vi "Get Processor Architecture.vi"() -> (0 "Processor Architecture":T1)   [LabVIEW 2020, in "binary_installation_tools.lvlib"]
uses:
  binary_installation_tools.lvlib
  <vilib>/registry/registry.llb/Registry RtKey.ctl
  <vilib>/registry/registry.llb/Registry SAM.ctl
  <vilib>/registry/registry.llb/Read Registry Value Simple STR.vi
  Processor Architecture.ctl
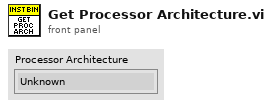
[diagram p1: front panel]
types:
  T1 = typedef "binary_installation_tools.lvlib/Processor Architecture.ctl" = enum16{"Unknown", "x86", "x64", "arm", "arm64"}
  T2 = typedef "Registry SAM.ctl" = enum32{"KEY_QUERY_VALUE", "KEY_SET_VALUE", "KEY_CREATE_SUB_KEY", "KEY_ENUMERATE_SUB_KEYS", "KEY_NOTIFY", "KEY_CREATE_LINK", "KEY_READ", "KEY_WRITE", "KEY_ALL_ACCESS", "KEY_READ | KEY_WRITE"}
  T3 = typedef "Registry RtKey.ctl" = enum32{"HKEY_CLASSES_ROOT", "HKEY_CURRENT_USER", "HKEY_LOCAL_MACHINE", "HKEY_USERS", "HKEY_PERFORMANCE_DATA", "HKEY_CURRENT_CONFIG", "HKEY_DYN_DATA"}
  T4 = typedef "Registry refnum.ctl" = refnum<k1>
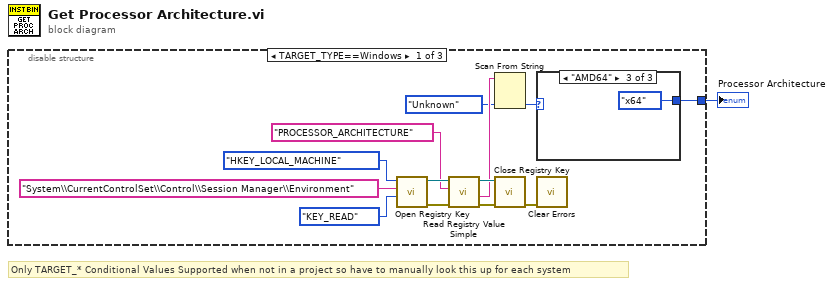
[diagram p0: block diagram]
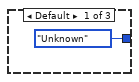
[diagram p2: hidden frame]
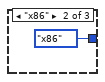
[diagram p3: hidden frame]
diagram:
  # "Only TARGET_* Conditional Values Supported when not in a project so have to manually look this up for each system"
  n1 = disable-structure shown="TARGET_TYPE==Windows" {
    disable-tunnel: [w2 _ _] -> w1
    frame condition #0 (active) {
      n2 = call <vilib>:"Open Registry Key.vi"("security access mask (KEY_READ | KEY_WRITE)"=Registry_SAM."KEY_READ", "subkey"="System\\CurrentControlSet\\Control\\Session Manager\\Environment", "root key (HKEY_LOCAL_MACHINE)"=Registry_RtKey."HKEY_LOCAL_MACHINE") -> ("error out"=w10:errorcluster, "refnum out"=w12:T4)  [unwired: 7 in]
      n3 = call-poly <vilib>:"Read Registry Value Simple.vi"("error in (no error)"=w10, "value"="PROCESSOR_ARCHITECTURE", "refnum"=w12) -> ("error out"=w8:errorcluster, "String/Binary data"=w5:string, "refnum out"=w7:T4)  [unwired: 3 in, 1 out]
      n4 = Scan From String(input string=w5, default 1=enum16{"Unknown", "x86", "AMD64"}."Unknown") -> (output 1=w3:enum16{"Unknown", "x86", "AMD64"})  [unwired: 3 in, 3 out]
      n5 = call <vilib>:"Close Registry Key.vi"("error in (no error)"=w8, "refnum"=w7) -> ("error out"=w6:errorcluster)  [unwired: 5 in]
      n6 = case shown="\"AMD64\"" w3 {
        tunnel: [Processor_Architecture."Unknown" ("Processor Architecture") Processor_Architecture."x86" ("Processor Architecture") Processor_Architecture."x64" ("Processor Architecture")] -> w2
        frame Default {
        }
        frame "x86" {
        }
        frame "AMD64" {
        }
      }
      n7 = call <vilib>:"Clear Errors.vi"("error in (no error)"=w6) -> ()  [unwired: 5 in, 2 out]
    }
    frame condition #1 {
    }
    frame condition #2 {
    }
  }
  "Processor Architecture" <- w1
